vi "Actor Core.vi"(8 "error in":errorcluster, 11 "File Logger in":refnum<class "File Logger.lvclass">) -> (0 "error out":errorcluster, 3 "Actor out":refnum<class "Actor.lvclass">)   [LabVIEW 2020, in "Logging.lvlib" / "File Logger.lvclass"]
doc: "(<B>Filename</B>: Actor Framework.lvlib:Actor.lvclass:Actor Core.vi)\n\nReceives messages to the actor, reacts to them, and initiates any error handling that may shut the actor down.\n\nDescendant classes may override this VI to append parallel tasks for the actor to complete while it handles messages. Overrides use the Call Parent Class Method node."
uses:
  File Logger.lvclass
  C:/Program Files (x86)/National Instruments/LabVIEW 2020/vi.lib/ActorFramework/Actor/Actor.lvclass
  <vilib>/ActorFramework/Actor/Actor.lvclass
  <vilib>/ActorFramework/Actor/Actor.lvclass/Actor.ctl
  <vilib>/ActorFramework/Message Enqueuer/Message Enqueuer.lvclass/Message Enqueuer.ctl
  <vilib>/ActorFramework/Message Enqueuer/Init from Existing Queue.vi
  <vilib>/ActorFramework/Message Enqueuer/Enqueue.vi
  <vilib>/ActorFramework/Stop Msg/Stop Msg.lvclass
  C:/Program Files (x86)/National Instruments/LabVIEW 2020/vi.lib/ActorFramework/Message/Message.lvclass
  <vilib>/ActorFramework/Message Priority Queue/Priority Enqueue.vi
  <vilib>/ActorFramework/Message Enqueuer/Message Enqueuer.lvclass
  Generic Logger/Generic Logger.lvclass
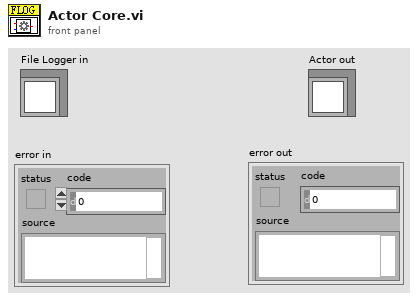
[diagram p1: front panel]
types:
  T1 = enum32{"Invalid", "Standard", "Closed", "Hidden", "Minimized", "Maximized"}
  T2 = cluster{"Stop event":refnum<user-event>, "Log Event":refnum<user-event>}
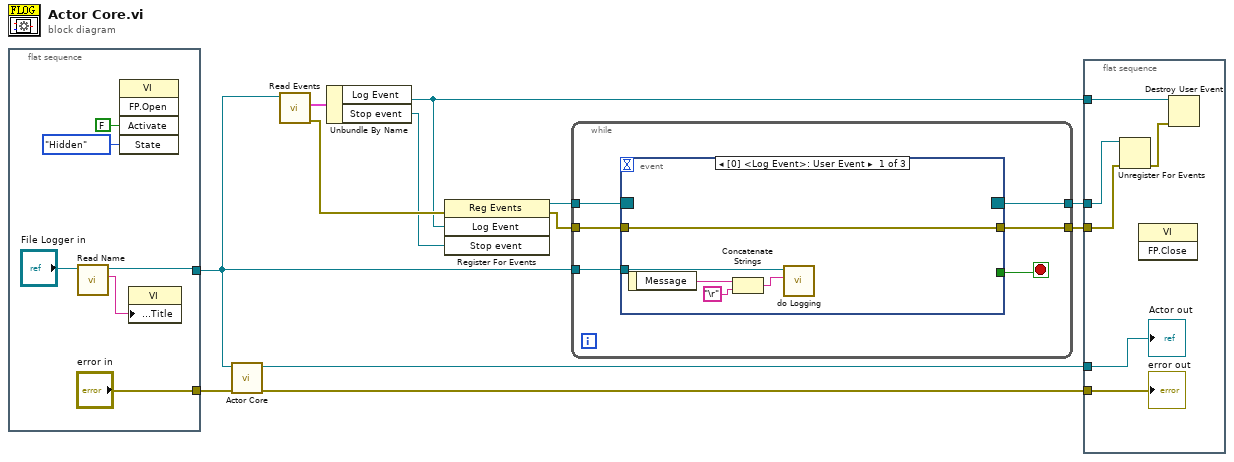
[diagram p0: block diagram]
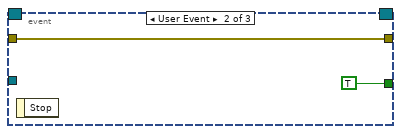
[diagram p2: hidden frame]
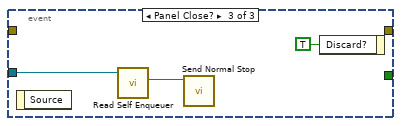
[diagram p3: hidden frame]
diagram:
  n1 = flat-sequence {
    tunnel: ["error in"] -> w11
    tunnel: [w15] -> w3
    frame #0 {
      n2 = call-dynamic "Read Name.vi"("Logger in"="File Logger in") -> ("Name"=w13:string, "Logger out"=w15:refnum<class "File Logger.lvclass">)  [unwired: 8 in, 1 out]
      n3 = invoke class="VI" method="FP.Open"("Activate"=FALSE ("Activate?"), "State"=T1."Hidden") -> ()  [unwired: 3 in, 5 out]
      n4 = property class="VI"("Front Panel.Title"=w13) -> ()  [unwired: 2 in, 2 out]
    }
  }
  n5 = call-parent "Actor Core.vi"("error in"=w11, "Actor in"=w3) -> ("error out"=w1:errorcluster, "Actor out"=w12:refnum<class "Actor.lvclass">)  [unwired: 8 in]
  n6 = call-dynamic "Read Events.vi"("Logger in"=w3) -> ("error out"=w7:errorcluster, "Events"=w8:T2)  [unwired: 8 in, 1 out]
  n7 = Unbundle By Name(w8) -> ("Log Event"=w5:refnum<user-event>, "Stop event"=w6:refnum<user-event>)
  n8 = register-events(error in=w7, w5, w6) -> (reference out=w10:refnum<event-registration>, error out=w9:errorcluster)  [unwired: 1 in]
  n9 = while {
    tunnel: w10 -> [w24]
    tunnel: w9 -> [w23]
    tunnel: [w21] -> w4
    tunnel: w3 -> [w20]
    tunnel: [w19] -> w2
    stop <- w22 stop-if-true
    n10 = event shown="[0] <Log Event>: User Event" {
      selector: w24 -> [_ _ _]
      dyn-events: [_ _ _] -> w21
      timeout: _ -> [_ _ _]
      tunnel: w23 -> [w29 w30 _]
      tunnel: [_ TRUE _] -> w22
      tunnel: w20 -> [w28 _ w33]
      tunnel: [w29 w30 _] -> w19
      event User Event {
        n11 = event-data() -> ("Message"=w27:string)  [unwired: 1 in]
        n12 = Concatenate Strings(w27, "\r") -> (w26:string)
        n13 = call-dynamic "do Logging.vi"("Content"=w26, "File Logger in"=w28) -> ()  [unwired: 8 in, 2 out]
      }
      event User Event {
        n14 = event-data() -> ()  [unwired: 1 in, 1 out]
      }
      event Panel Close? {
        n15 = event-data() -> ()  [unwired: 1 in, 1 out]
        n16 = call <vilib>:"Read Self Enqueuer.vi"("Actor"=w33) -> ("Self Enqueuer"=w34:refnum<class "Message Enqueuer.lvclass">)  [unwired: 10 in]
        n17 = call <vilib>:"Send Normal Stop.vi"("Message Enqueuer"=w34) -> ()  [unwired: 10 in, 1 out]
        n18 = event-data("Discard?"=TRUE) -> ()  [unwired: 1 in, 1 out]
      }
    }
  }
  n19 = flat-sequence {
    tunnel: w12 -> [w40]
    tunnel: w5 -> [w38]
    tunnel: w4 -> [w37]
    tunnel: w2 -> [w36]
    tunnel: w1 -> [w35]
    frame #0 {
      n20 = Unregister For Events(event registration refnum=w37, error in=w36) -> (error out=w39:errorcluster)
      n21 = invoke class="VI" method="FP.Close"() -> ()  [unwired: 3 in, 3 out]
      n22 = Destroy User Event(user event=w38, error in=w39) -> ()  [unwired: 1 out]
      "error out" <- w35
      "Actor out" <- w40
    }
  }
